vi "MotorControllerGUI_xiang_test.vi"() -> ()   [LabVIEW 2017]
uses:
  Newport.CONEXCC.CommandInterface
  location.ctl
panel:
  in  "stop":bool
  in  "Direction Pad":T1={"right+"=FALSE, "right"=FALSE, "left"=FALSE, "left+"=FALSE, "up"=FALSE, "up+"=FALSE, "down+"=FALSE, "down"=FALSE, "motor stop"=FALSE, "Velocity (mm/s)"=2.0, "Step (mm)"=0.1}
  in  "Radius Limit (mm)":dbl=5.0
  out "Location plot":cluster{dbl[], dbl[]}[](graph)
  out "Current Location":T2 {"Position"."Position Y" format="%#.3f"; "Position"."Position X" format="%#.3f"}
  out "Key Move?":bool
  out "errstring":string
  out "errstring 2":string
  out "PA_Set":i32
  out "PA_Set 2":i32
  out "error out":errorcluster
  out "X Motor ID":string
  out "Y Motor ID":string
  in  "Y COM port":string="COM3"
  in  "X COM port":string="COM4"
  out "Center location":T2 {"Position"."Position Y" format="%#.3f"; "Position"."Position X" format="%#.3f"}
  out "Circle":cluster{dbl[], dbl[]}
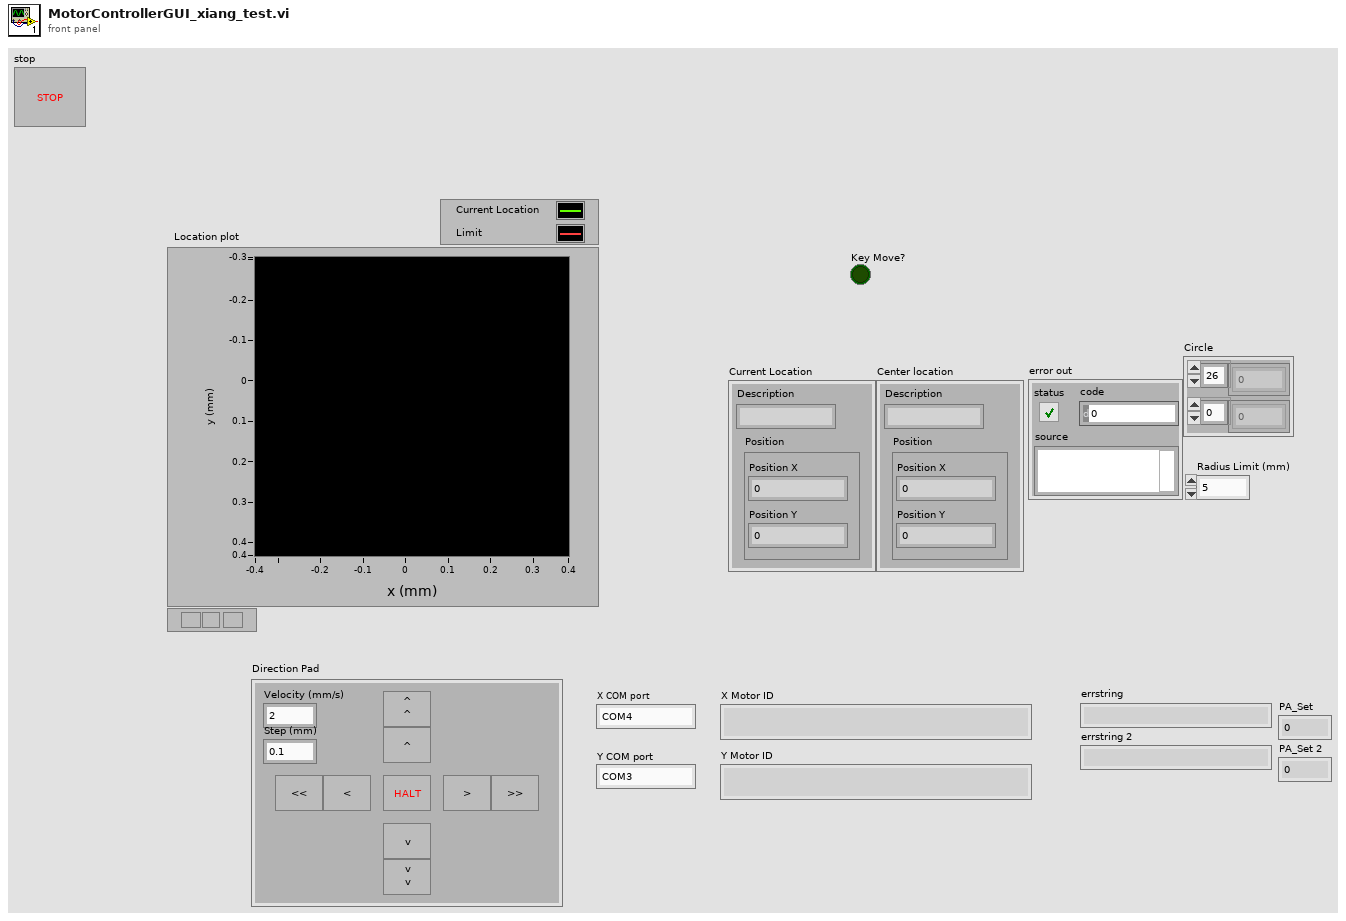
[diagram p1: front panel]
types:
  T1 = cluster{"right+":bool, "right":bool, "left":bool, "left+":bool, "up":bool, "up+":bool, "down+":bool, "down":bool, "motor stop":bool, "Velocity (mm/s)":dbl, "Step (mm)":dbl}
  T2 = typedef "location.ctl" = cluster{"Description":string, "Position":cluster{"Position X":dbl, "Position Y":dbl}}
  T3 = typedef "eventvkey.ctl" = enum16{"ASCII", "Enter", "Return", "Shift", "Ctrl", "Alt", "Cmd", "Opt", "Caps", "NumLock", "Clear", "Break", "Up", "Down", "Left", "Right", "Insert", "Delete", "Home", "End", "PageUp", "PageDown", "Escape", "Help", "Pause", "ScrollLock", "F1", "F2", "F3", "F4", "F5", "F6", "F7", "F8", "F9", "F10", "F11", "F12", "F13", "F14", "F15", "F16", "F17", "F18", "F19", "F20", "F21", "F22", "F23", "F24", "Play", "VolumeUp", "VolumeDown", "Mute", "Two Byte Char"}
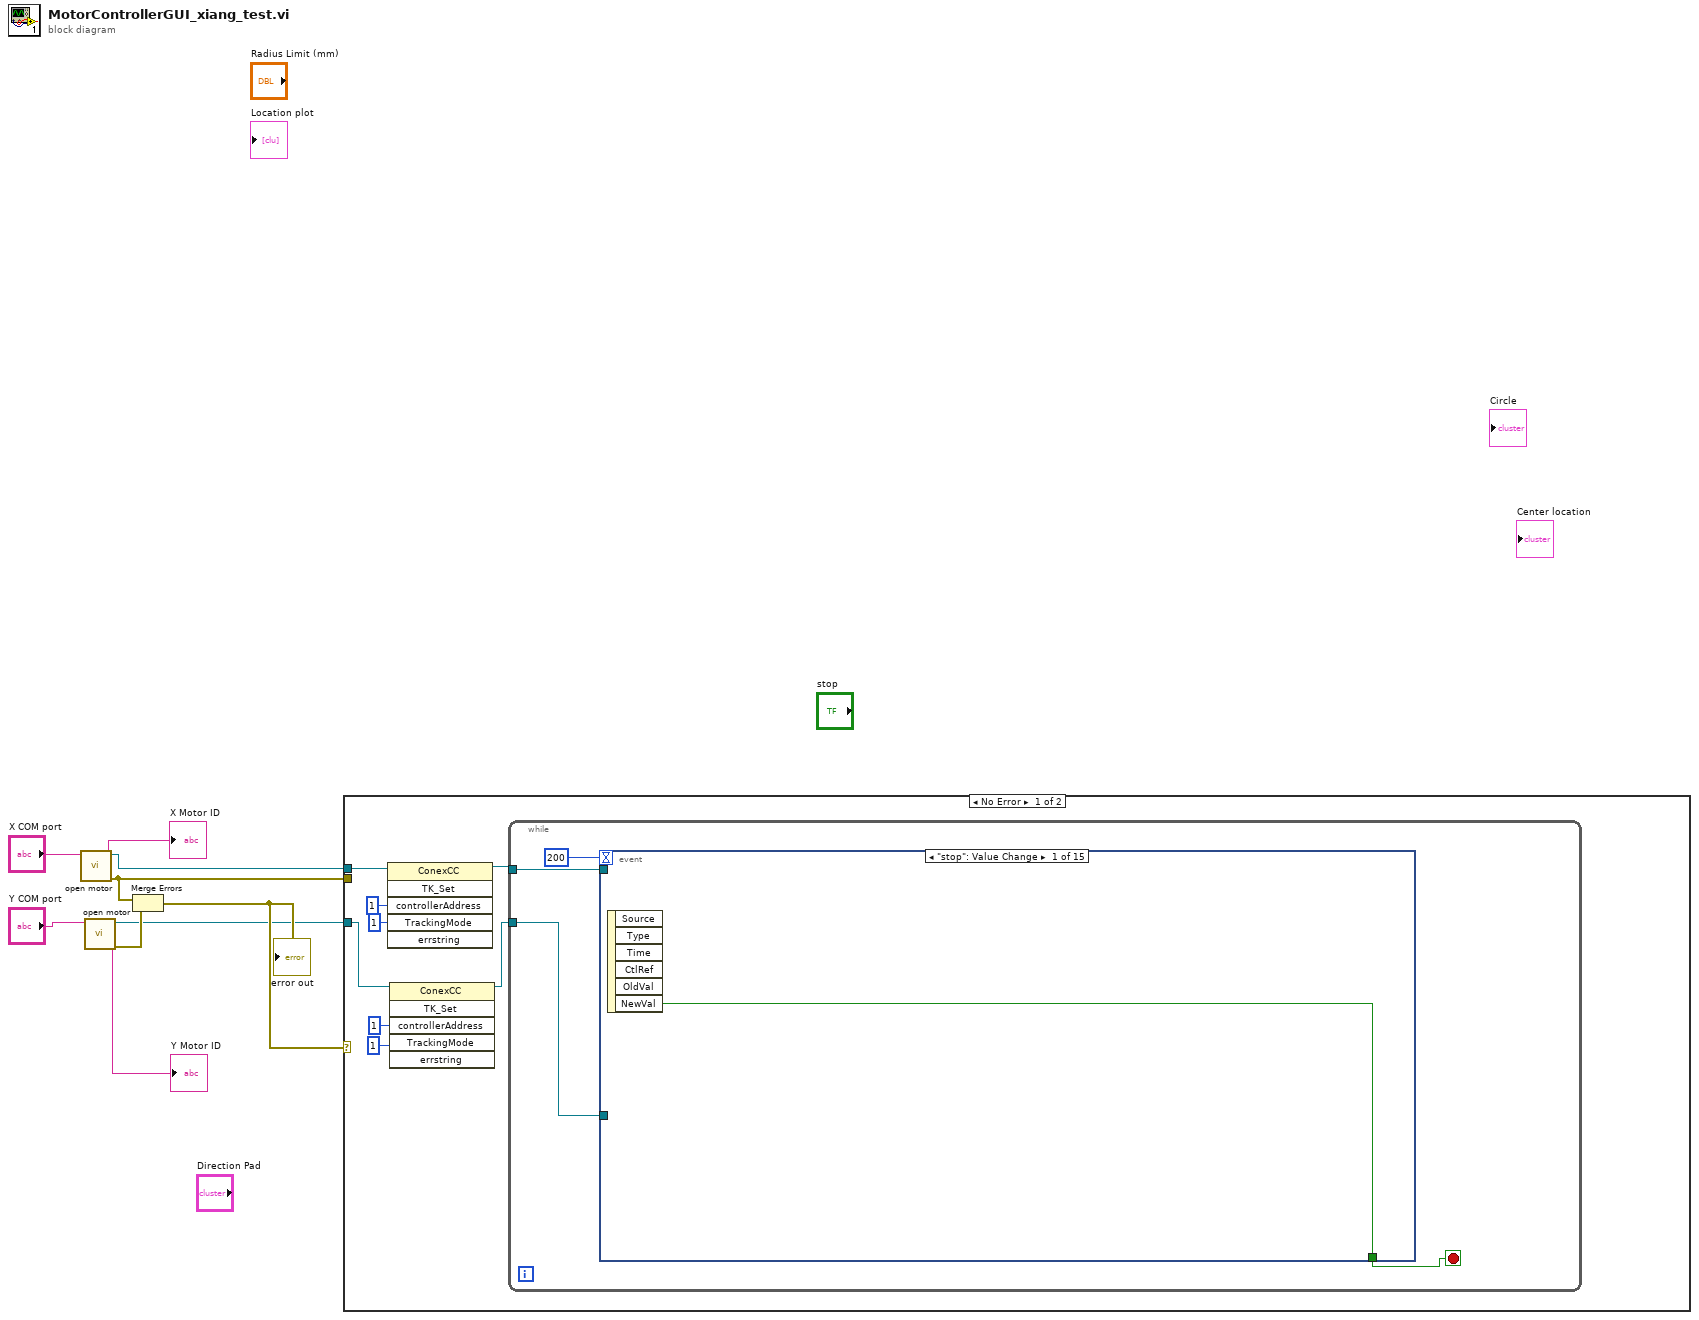
[diagram p0: block diagram]
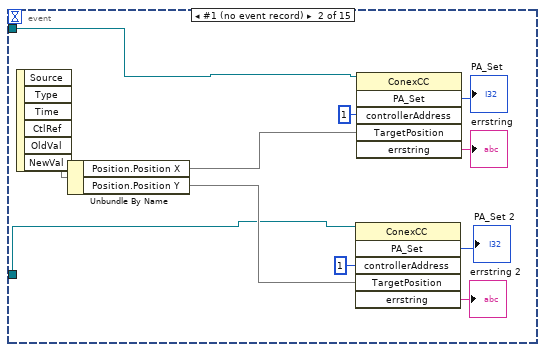
[diagram p2: hidden frame]
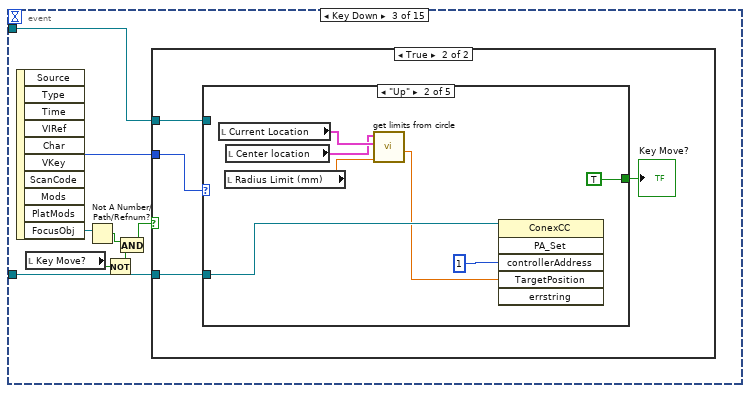
[diagram p3: hidden frame]
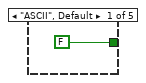
[diagram p5: hidden frame]
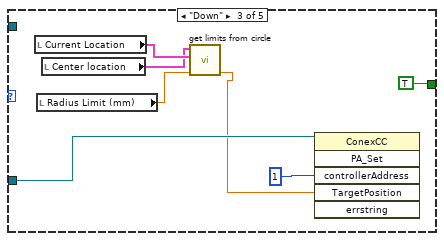
[diagram p6: hidden frame]
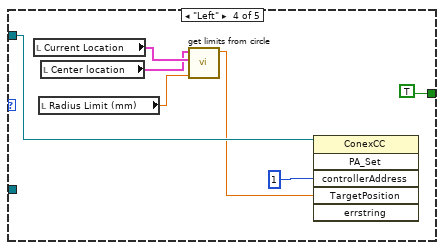
[diagram p7: hidden frame]
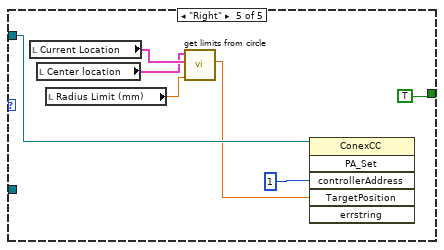
[diagram p8: hidden frame]
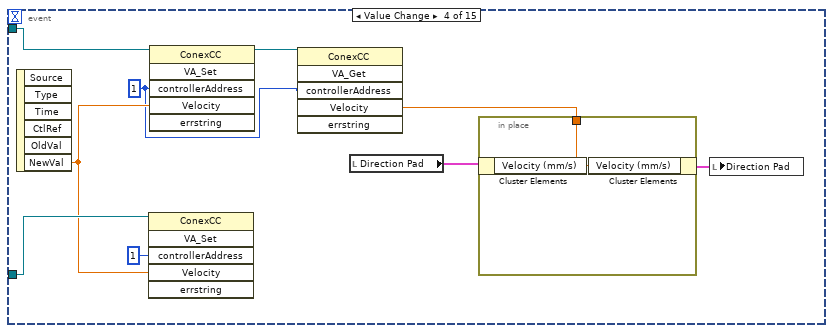
[diagram p9: hidden frame]
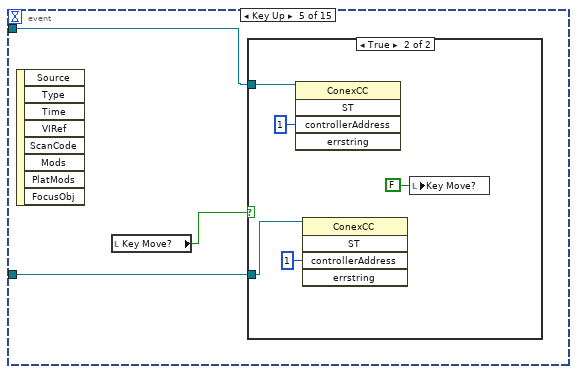
[diagram p10: hidden frame]
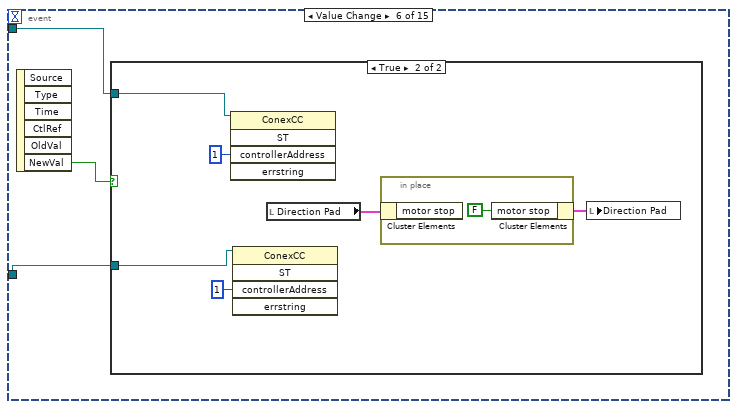
[diagram p12: hidden frame]
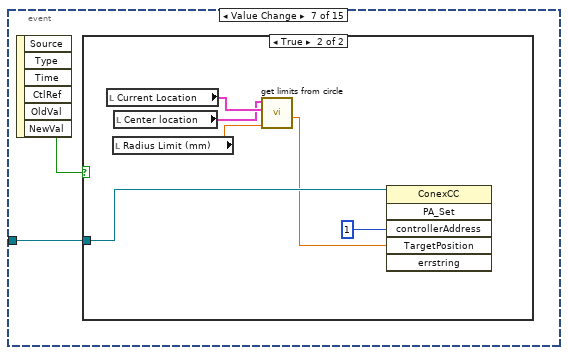
[diagram p14: hidden frame]
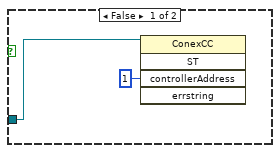
[diagram p15: hidden frame]
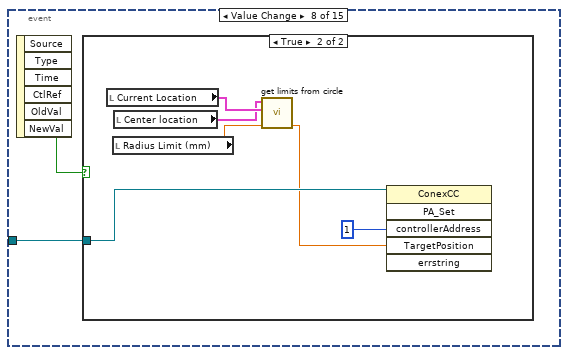
[diagram p16: hidden frame]
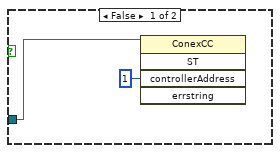
[diagram p17: hidden frame]
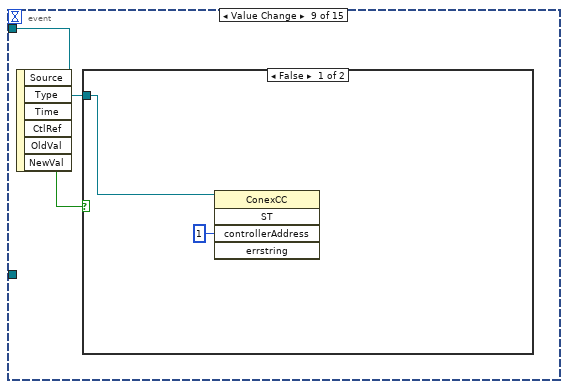
[diagram p18: hidden frame]
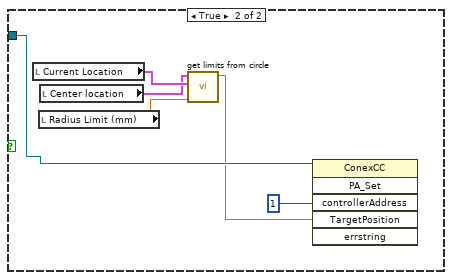
[diagram p19: hidden frame]
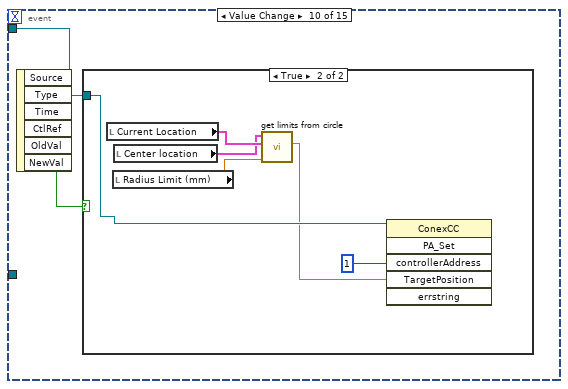
[diagram p20: hidden frame]
diagram:
  n1 = call "open motor.vi"("COM port"="X COM port") -> ("error out"=w3:errorcluster, "Motor ID"=→"X Motor ID":string, "CONEX_CC"=w2:refnum<k24>)  [unwired: 8 in]
  n2 = call "open motor.vi"("COM port"="Y COM port") -> ("error out"=w5:errorcluster, "Motor ID"=→"Y Motor ID":string, "CONEX_CC"=w1:refnum<k24>)  [unwired: 8 in]
  n3 = Merge Errors(w3, w5) -> (w4:errorcluster)
  "error out" <- w4
  n4 = case shown="No Error" w4 {
    tunnel: w3 -> [_ _]
    tunnel: w2 -> [w11 _]
    tunnel: w1 -> [w15 _]
    frame No Error {
      n5 = invoke class="ConexCC" method="TK_Set"(reference=w11, "controllerAddress"=1, "TrackingMode"=1) -> (reference out=w10:refnum<k24>)  [unwired: 3 in, 5 out]
      n6 = invoke class="ConexCC" method="TK_Set"(reference=w15, "controllerAddress"=1, "TrackingMode"=1) -> (reference out=w14:refnum<k24>)  [unwired: 3 in, 5 out]
      n7 = while {
        tunnel: w10 -> [w21]
        tunnel: w14 -> [w20]
        stop <- w18 stop-if-true
        n8 = event shown="[0] \"stop\": Value Change" {
          selector: _ -> [_ _ _ _ _ _ _ _ _ _ _ _ _ _ _]
          dyn-events: _ -> [_ _ _ _ _ _ _ _ _ _ _ _ _ _ _]
          timeout: 200 -> [_ _ _ _ _ _ _ _ _ _ _ _ _ _ _]
          tunnel: [w22 _ _ _ _ _ _ _ _ _ _ _ _ _ _] -> w18
          tunnel: w21 -> [_ w24 w39 w83 w86 w94 _ _ w123 w133 _ _ w175 w191 w219]
          tunnel: w20 -> [_ w23 w38 w82 w85 w93 w103 w113 _ _ w143 w159 _ _ w218]
          event "stop": Value Change {
            n9 = event-data() -> ("NewVal"=w22:bool)  [unwired: 1 in, 5 out]
          }
          event #1 (no event record) {
            n10 = event-data() -> ("NewVal"=w33)  [unwired: 1 in, 5 out]
            n11 = Unbundle By Name(w33) -> ("Position.Position X"=w32, "Position.Position Y"=w31)
            n12 = invoke class="ConexCC" method="PA_Set"(reference=w23, "controllerAddress"=1, "TargetPosition"=w31) -> ("PA_Set"=→"PA_Set 2":i32, "errstring"=→"errstring 2":string)  [unwired: 3 in, 4 out]
            n13 = invoke class="ConexCC" method="PA_Set"(reference=w24, "controllerAddress"=1, "TargetPosition"=w32) -> ("PA_Set"=→"PA_Set":i32, "errstring"=→"errstring":string)  [unwired: 3 in, 4 out]
          }
          event Key Down {
            n14 = event-data() -> ("VKey"=w40:T3, "FocusObj"=w41:refnum<vi>)  [unwired: 1 in, 8 out]
            n15 = local read "Key Move?"() -> (w36:bool)
            n16 = Not A Number/Path/Refnum?(number/path/refnum=w41) -> (NaN/Path/Refnum?=w37:bool)
            n17 = Not(x=w36) -> (.not. x?=w35:bool)
            n18 = And(x=w37, y=w35) -> (x .and. y?=w34:bool)
            n19 = case shown="True" w34 {
              tunnel: w40 -> [_ w45]
              tunnel: w39 -> [_ w43]
              tunnel: w38 -> [_ w42]
              frame False {
              }
              frame True {
                n20 = case shown="\"Up\"" w45 {
                  tunnel: [FALSE TRUE TRUE TRUE TRUE] -> w44
                  tunnel: w43 -> [_ _ _ w63 w70]
                  tunnel: w42 -> [_ w52 w56 _ _]
                  frame "ASCII", Default {
                  }
                  frame "Up" {
                    n21 = local read "Current Location"() -> (w50:T2)
                    n22 = local read "Radius Limit (mm)"() -> (w48:dbl)
                    n23 = local read "Center location"() -> (w49:T2)
                    n24 = call "get limits from circle.vi"("Radius"=w48, "Current Location"=w50, "Center location"=w49) -> ("Ymin given x"=w47:dbl)  [unwired: 5 in, 3 out]
                    n25 = invoke class="ConexCC" method="PA_Set"(reference=w52, "controllerAddress"=1, "TargetPosition"=w47) -> ()  [unwired: 3 in, 6 out]
                  }
                  frame "Down" {
                    n26 = local read "Current Location"() -> (w58:T2)
                    n27 = local read "Radius Limit (mm)"() -> (w55:dbl)
                    n28 = local read "Center location"() -> (w57:T2)
                    n29 = call "get limits from circle.vi"("Radius"=w55, "Current Location"=w58, "Center location"=w57) -> ("Ymax given x"=w54:dbl)  [unwired: 5 in, 3 out]
                    n30 = invoke class="ConexCC" method="PA_Set"(reference=w56, "controllerAddress"=1, "TargetPosition"=w54) -> ()  [unwired: 3 in, 6 out]
                  }
                  frame "Left" {
                    n31 = local read "Current Location"() -> (w65:T2)
                    n32 = local read "Radius Limit (mm)"() -> (w61:dbl)
                    n33 = local read "Center location"() -> (w64:T2)
                    n34 = call "get limits from circle.vi"("Radius"=w61, "Current Location"=w65, "Center location"=w64) -> ("Xmin given y"=w62:dbl)  [unwired: 5 in, 3 out]
                    n35 = invoke class="ConexCC" method="PA_Set"(reference=w63, "controllerAddress"=1, "TargetPosition"=w62) -> ()  [unwired: 3 in, 6 out]
                  }
                  frame "Right" {
                    n36 = local read "Current Location"() -> (w72:T2)
                    n37 = local read "Center location"() -> (w71:T2)
                    n38 = local read "Radius Limit (mm)"() -> (w69:dbl)
                    n39 = call "get limits from circle.vi"("Radius"=w69, "Current Location"=w72, "Center location"=w71) -> ("Xmax given y"=w68:dbl)  [unwired: 5 in, 3 out]
                    n40 = invoke class="ConexCC" method="PA_Set"(reference=w70, "controllerAddress"=1, "TargetPosition"=w68) -> ()  [unwired: 3 in, 6 out]
                  }
                }
                "Key Move?" <- w44
              }
            }
          }
          event "Direction Pad.Velocity (mm/s)": Value Change {
            w75 = 1 ("controllerAddress")
            n41 = event-data() -> ("NewVal"=w81:dbl)  [unwired: 1 in, 5 out]
            n42 = invoke class="ConexCC" method="VA_Set"(reference=w82, "controllerAddress"=1, "Velocity"=w81) -> ()  [unwired: 3 in, 6 out]
            n43 = invoke class="ConexCC" method="VA_Set"(reference=w83, "controllerAddress"=w75, "Velocity"=w81) -> (reference out=w79:refnum<k24>)  [unwired: 3 in, 5 out]
            n44 = invoke class="ConexCC" method="VA_Get"(reference=w79, "controllerAddress"=w75) -> ("Velocity"=w77:dbl)  [unwired: 4 in, 5 out]
            n45 = local read "Direction Pad"() -> (w78:T1)
            n46 = in-place {
              in-place-border: w77 -> [w84]
              n47 = in-place-cluster #1(w78) -> ()  [unwired: 1 out]
              n48 = in-place-cluster #1("Velocity (mm/s)"=w84) -> (w76:T1)
            }
            n49 = local write "Direction Pad"(w76) -> ()
          }
          event Key Up {
            n50 = event-data() -> ()  [unwired: 1 in, 8 out]
            n51 = local read "Key Move?"() -> (w87:bool)
            n52 = case shown="True" w87 {
              tunnel: w86 -> [_ w92]
              tunnel: w85 -> [_ w90]
              frame False {
              }
              frame True {
                n53 = invoke class="ConexCC" method="ST"(reference=w92, "controllerAddress"=1) -> ()  [unwired: 3 in, 5 out]
                n54 = invoke class="ConexCC" method="ST"(reference=w90, "controllerAddress"=1) -> ()  [unwired: 3 in, 5 out]
                n55 = local write "Key Move?"(FALSE ("Key Move?")) -> ()
              }
            }
          }
          event "Direction Pad.motor stop": Value Change {
            n56 = event-data() -> ("NewVal"=w95:bool)  [unwired: 1 in, 5 out]
            n57 = case shown="True" w95 {
              tunnel: w94 -> [_ w101]
              tunnel: w93 -> [_ w100]
              frame False {
              }
              frame True {
                n58 = invoke class="ConexCC" method="ST"(reference=w101, "controllerAddress"=1) -> ()  [unwired: 3 in, 5 out]
                n59 = invoke class="ConexCC" method="ST"(reference=w100, "controllerAddress"=1) -> ()  [unwired: 3 in, 5 out]
                n60 = local read "Direction Pad"() -> (w97:T1)
                n61 = in-place {
                  n62 = in-place-cluster #2(w97) -> ()  [unwired: 1 out]
                  n63 = in-place-cluster #2("motor stop"=FALSE) -> (w96:T1)
                }
                n64 = local write "Direction Pad"(w96) -> ()
              }
            }
          }
          event "Direction Pad.up+": Value Change {
            n65 = event-data() -> ("NewVal"=w104:bool)  [unwired: 1 in, 5 out]
            n66 = case shown="True" w104 {
              tunnel: w103 -> [w105 w108]
              frame False {
                n67 = invoke class="ConexCC" method="ST"(reference=w105, "controllerAddress"=1) -> ()  [unwired: 3 in, 5 out]
              }
              frame True {
                n68 = local read "Current Location"() -> (w112:T2)
                n69 = local read "Radius Limit (mm)"() -> (w110:dbl)
                n70 = local read "Center location"() -> (w111:T2)
                n71 = call "get limits from circle.vi"("Radius"=w110, "Current Location"=w112, "Center location"=w111) -> ("Ymin given x"=w107:dbl)  [unwired: 5 in, 3 out]
                n72 = invoke class="ConexCC" method="PA_Set"(reference=w108, "controllerAddress"=1, "TargetPosition"=w107) -> ()  [unwired: 3 in, 6 out]
              }
            }
          }
          event "Direction Pad.down+": Value Change {
            n73 = event-data() -> ("NewVal"=w114:bool)  [unwired: 1 in, 5 out]
            n74 = case shown="True" w114 {
              tunnel: w113 -> [w115 w118]
              frame False {
                n75 = invoke class="ConexCC" method="ST"(reference=w115, "controllerAddress"=1) -> ()  [unwired: 3 in, 5 out]
              }
              frame True {
                n76 = local read "Current Location"() -> (w122:T2)
                n77 = local read "Radius Limit (mm)"() -> (w120:dbl)
                n78 = local read "Center location"() -> (w121:T2)
                n79 = call "get limits from circle.vi"("Radius"=w120, "Current Location"=w122, "Center location"=w121) -> ("Ymax given x"=w117:dbl)  [unwired: 5 in, 3 out]
                n80 = invoke class="ConexCC" method="PA_Set"(reference=w118, "controllerAddress"=1, "TargetPosition"=w117) -> ()  [unwired: 3 in, 6 out]
              }
            }
          }
          event "Direction Pad.left+": Value Change {
            n81 = event-data() -> ("NewVal"=w124:bool)  [unwired: 1 in, 5 out]
            n82 = case shown="False" w124 {
              tunnel: w123 -> [w125 w128]
              frame False {
                n83 = invoke class="ConexCC" method="ST"(reference=w125, "controllerAddress"=1) -> ()  [unwired: 3 in, 5 out]
              }
              frame True {
                n84 = local read "Current Location"() -> (w132:T2)
                n85 = local read "Radius Limit (mm)"() -> (w130:dbl)
                n86 = local read "Center location"() -> (w131:T2)
                n87 = call "get limits from circle.vi"("Radius"=w130, "Current Location"=w132, "Center location"=w131) -> ("Xmin given y"=w127:dbl)  [unwired: 5 in, 3 out]
                n88 = invoke class="ConexCC" method="PA_Set"(reference=w128, "controllerAddress"=1, "TargetPosition"=w127) -> ()  [unwired: 3 in, 6 out]
              }
            }
          }
          event "Direction Pad.right+": Value Change {
            n89 = event-data() -> ("NewVal"=w134:bool)  [unwired: 1 in, 5 out]
            n90 = case shown="True" w134 {
              tunnel: w133 -> [w135 w138]
              frame False {
                n91 = invoke class="ConexCC" method="ST"(reference=w135, "controllerAddress"=1) -> ()  [unwired: 3 in, 5 out]
              }
              frame True {
                n92 = local read "Current Location"() -> (w142:T2)
                n93 = local read "Radius Limit (mm)"() -> (w140:dbl)
                n94 = local read "Center location"() -> (w141:T2)
                n95 = call "get limits from circle.vi"("Radius"=w140, "Current Location"=w142, "Center location"=w141) -> ("Xmax given y"=w137:dbl)  [unwired: 5 in, 3 out]
                n96 = invoke class="ConexCC" method="PA_Set"(reference=w138, "controllerAddress"=1, "TargetPosition"=w137) -> ()  [unwired: 3 in, 6 out]
              }
            }
          }
          event "Direction Pad.up": Value Change {
            n97 = event-data() -> ("NewVal"=w144:bool)  [unwired: 1 in, 5 out]
            n98 = case shown="True" w144 {
              tunnel: w143 -> [_ w154]
              frame False {
              }
              frame True {
                n99 = local read "Current Location"() -> (w155:T2)
                n100 = local read "Radius Limit (mm)"() -> (w156:dbl)
                n101 = local read "Center location"() -> (w157:T2)
                n102 = local read "Direction Pad"() -> (w151:T1)
                n103 = Unbundle By Name(w155) -> ("Position.Position Y"=w153:dbl)
                n104 = Unbundle By Name(w151) -> ("Step (mm)"=w150:dbl)
                n105 = in-place {
                  n106 = in-place-cluster #3(w151) -> ()  [unwired: 1 out]
                  n107 = in-place-cluster #3("up"=FALSE ("motor stop")) -> (w152:T1)
                }
                n108 = call "get limits from circle.vi"("Radius"=w156, "Current Location"=w155, "Center location"=w157) -> ("Ymax given x"=w146:dbl, "Ymin given x"=w147:dbl)  [unwired: 5 in, 2 out]
                n109 = Subtract(x=w153, y=w150) -> (x-y=w148:dbl)
                n110 = In Range and Coerce(upper limit=w146, x=w148, lower limit=w147) -> (coerced(x)=w145:dbl)  [unwired: 1 out]
                n111 = local write "Direction Pad"(w152) -> ()
                n112 = invoke class="ConexCC" method="PA_Set"(reference=w154, "controllerAddress"=1, "TargetPosition"=w145) -> ()  [unwired: 3 in, 6 out]
              }
            }
          }
          event "Direction Pad.down": Value Change {
            n113 = event-data() -> ("NewVal"=w160:bool)  [unwired: 1 in, 5 out]
            n114 = case shown="True" w160 {
              tunnel: w159 -> [_ w170]
              frame False {
              }
              frame True {
                n115 = local read "Current Location"() -> (w171:T2)
                n116 = local read "Radius Limit (mm)"() -> (w172:dbl)
                n117 = local read "Center location"() -> (w173:T2)
                n118 = local read "Direction Pad"() -> (w167:T1)
                n119 = Unbundle By Name(w171) -> ("Position.Position Y"=w169:dbl)
                n120 = Unbundle By Name(w167) -> ("Step (mm)"=w166:dbl)
                n121 = in-place {
                  n122 = in-place-cluster #4(w167) -> ()  [unwired: 1 out]
                  n123 = in-place-cluster #4("down"=FALSE ("motor stop")) -> (w168:T1)
                }
                n124 = call "get limits from circle.vi"("Radius"=w172, "Current Location"=w171, "Center location"=w173) -> ("Ymax given x"=w162:dbl, "Ymin given x"=w163:dbl)  [unwired: 5 in, 2 out]
                n125 = Add(x=w169, y=w166) -> (x+y=w164:dbl)
                n126 = In Range and Coerce(upper limit=w162, x=w164, lower limit=w163) -> (coerced(x)=w161:dbl)  [unwired: 1 out]
                n127 = local write "Direction Pad"(w168) -> ()
                n128 = invoke class="ConexCC" method="PA_Set"(reference=w170, "controllerAddress"=1, "TargetPosition"=w161) -> ()  [unwired: 3 in, 6 out]
              }
            }
          }
          event "Direction Pad.left": Value Change {
            n129 = event-data() -> ("NewVal"=w176:bool)  [unwired: 1 in, 5 out]
            n130 = case shown="True" w176 {
              tunnel: w175 -> [_ w186]
              frame False {
              }
              frame True {
                n131 = local read "Current Location"() -> (w187:T2)
                n132 = local read "Radius Limit (mm)"() -> (w188:dbl)
                n133 = local read "Center location"() -> (w189:T2)
                n134 = local read "Direction Pad"() -> (w184:T1)
                n135 = Unbundle By Name(w187) -> ("Position.Position X"=w177:dbl)
                n136 = Unbundle By Name(w184) -> ("Step (mm)"=w183:dbl)
                n137 = in-place {
                  n138 = in-place-cluster #5(w184) -> ()  [unwired: 1 out]
                  n139 = in-place-cluster #5("left"=FALSE ("motor stop")) -> (w185:T1)
                }
                n140 = call "get limits from circle.vi"("Radius"=w188, "Current Location"=w187, "Center location"=w189) -> ("Xmax given y"=w178:dbl, "Xmin given y"=w179:dbl)  [unwired: 5 in, 2 out]
                n141 = Subtract(x=w177, y=w183) -> (x-y=w181:dbl)
                n142 = In Range and Coerce(upper limit=w178, x=w181, lower limit=w179) -> (coerced(x)=w180:dbl)  [unwired: 1 out]
                n143 = local write "Direction Pad"(w185) -> ()
                n144 = invoke class="ConexCC" method="PA_Set"(reference=w186, "controllerAddress"=1, "TargetPosition"=w180) -> ()  [unwired: 3 in, 6 out]
              }
            }
          }
          event "Direction Pad.right": Value Change {
            n145 = event-data() -> ("NewVal"=w192:bool)  [unwired: 1 in, 5 out]
            n146 = case shown="True" w192 {
              tunnel: w191 -> [_ w202]
              frame False {
              }
              frame True {
                n147 = local read "Current Location"() -> (w203:T2)
                n148 = local read "Radius Limit (mm)"() -> (w204:dbl)
                n149 = local read "Center location"() -> (w205:T2)
                n150 = local read "Direction Pad"() -> (w200:T1)
                n151 = Unbundle By Name(w203) -> ("Position.Position X"=w193:dbl)
                n152 = Unbundle By Name(w200) -> ("Step (mm)"=w199:dbl)
                n153 = in-place {
                  n154 = in-place-cluster #6(w200) -> ()  [unwired: 1 out]
                  n155 = in-place-cluster #6("right"=FALSE ("motor stop")) -> (w201:T1)
                }
                n156 = call "get limits from circle.vi"("Radius"=w204, "Current Location"=w203, "Center location"=w205) -> ("Xmax given y"=w194:dbl, "Xmin given y"=w195:dbl)  [unwired: 5 in, 2 out]
                n157 = Add(x=w193, y=w199) -> (x+y=w197:dbl)
                n158 = In Range and Coerce(upper limit=w194, x=w197, lower limit=w195) -> (coerced(x)=w196:dbl)  [unwired: 1 out]
                n159 = local write "Direction Pad"(w201) -> ()
                n160 = invoke class="ConexCC" method="PA_Set"(reference=w202, "controllerAddress"=1, "TargetPosition"=w196) -> ()  [unwired: 3 in, 6 out]
              }
            }
          }
          event Timeout {
            n161 = event-data() -> ()  [unwired: 1 in, 3 out]
            n162 = invoke class="ConexCC" method="TP"(reference=w219, "controllerAddress"=1) -> ("CurrentPosition"=w208:dbl)  [unwired: 4 in, 5 out]
            n163 = invoke class="ConexCC" method="TP"(reference=w218, "controllerAddress"=1) -> ("CurrentPosition"=w207:dbl)  [unwired: 4 in, 5 out]
            n164 = Build Array(w208) -> (w214:dbl[])
            n165 = Build Array(w207) -> (w215:dbl[])
            n166 = local read "Current Location"() -> (w209:T2)
            n167 = Bundle By Name(cluster=w209, "Position.Position X"=w208, "Position.Position Y"=w207) -> (→"Current Location":T2)
            n168 = Bundle(w214, w215) -> (w213:cluster{dbl[], dbl[]})  [unwired: 1 in]
            n169 = local read "Circle"() -> (w211:cluster{dbl[], dbl[]})
            n170 = Build Array(w213, w211) -> (w212:cluster{dbl[], dbl[]}[])
            n171 = local write "Location plot"(w212) -> ()
          }
        }
      }
    }
    frame Error {
    }
  }
